vi "Trig_TimeCheck.vi"(8 "error in (no error)":errorcluster, 11 "cmd":T1) -> (0 "error out":errorcluster)   [LabVIEW 2019]
uses:
  cmd_offtimecheck.ctl
  _ctrl/system-status.ctl
  _ctrl/rw.ctl
  _ctrl/init-r-stop.ctl
  Durability/common/Global_params.vi
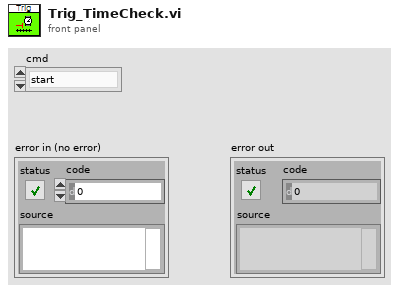
[diagram p1: front panel]
types:
  T1 = typedef "cmd_offtimecheck.ctl" = enum16{"start", "check", "init"}
  T2 = typedef "rw.ctl" = enum16{"read", "write"}
  T3 = typedef "system-status.ctl" = enum16{"Initial", "Update", "Clear", "Read"}
  T4 = typedef "init-r-stop.ctl" = enum16{"ini", "read", "stop"}
  T5 = typedef "cap_config.ctl" = cluster{"Test Mode":T6, "ON time[ms]":dbl, "OFF time[ms]":dbl, "1. 작동시간[분]":dbl, "2. 미작동시간[분]":dbl, "3. 작동시간[분]":dbl, "level[V]":dbl, "duty":dbl, "Freq":dbl, "Voltage+[V]":dbl, "Voltage-[V]":dbl, "Current+[A]":dbl, "Current-[A]":dbl, "출력전압[V]":dbl, "출력전류[A]":dbl, "OVP Level":dbl, "OCP Level":dbl, "Time Div":u16, "Record Len":i32, "방전 기준[V]":dbl, "Repeate (Each Ch)":u32, "Cycle[N]":u32, "작동간격[분]":dbl, "TrigPos[%]":dbl, "시험시간[분]":dbl}
  T6 = typedef "시험모드선택.ctl" = enum16{"6.3.1 온도방치 시험", "6.3.2 저온 작동/방치 시험", "6.3.3 고온 작동/방치 시험", "6.3.4 온도 싸이클 시험", "6.3.6 온습도 싸이클 시험", "6.3.7 고온고습 방치", "6.3.8 결로 시험", "6.3.9 빙결시험", "6.3.11.1 작동가진", "6.3.12 충격시험"}
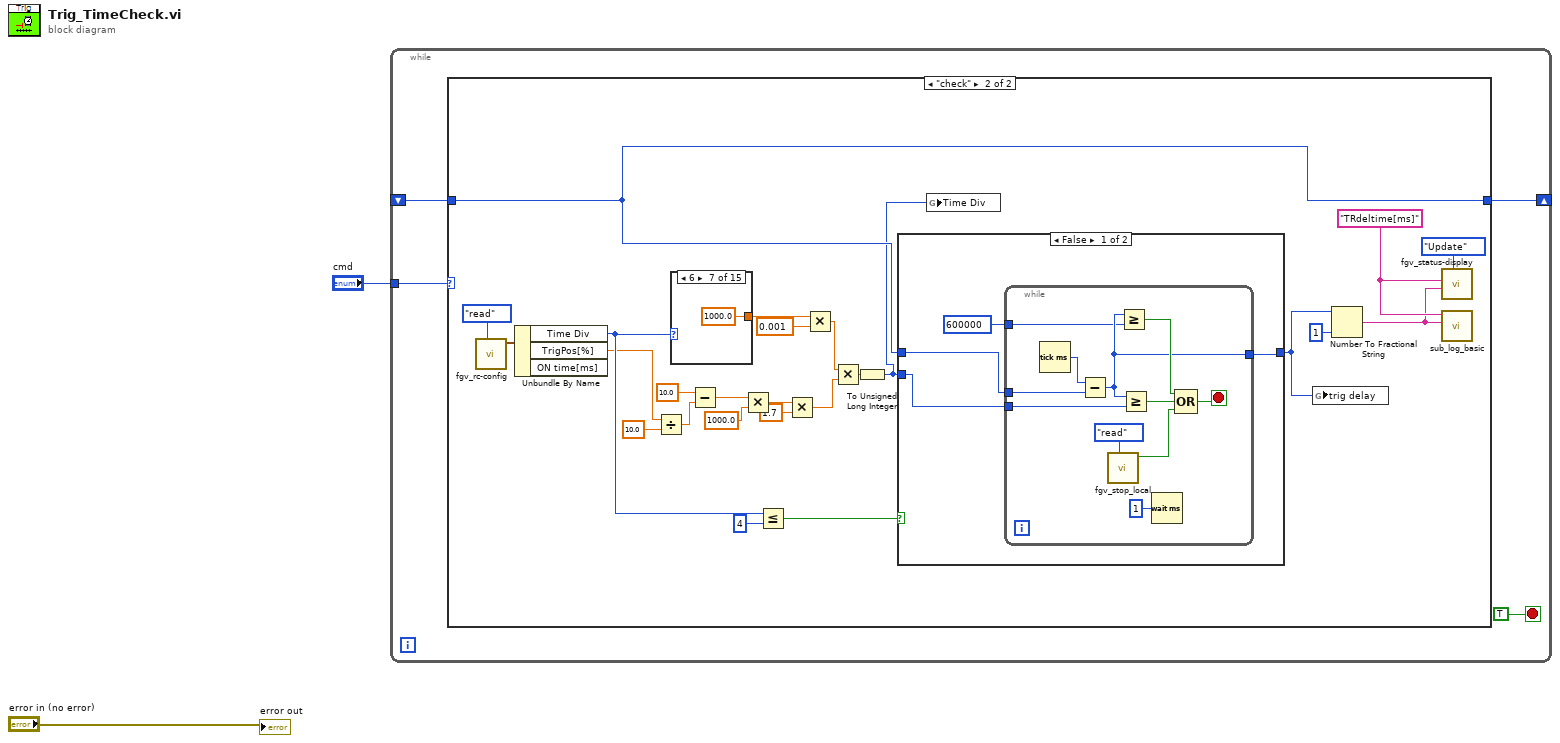
[diagram p0: block diagram]
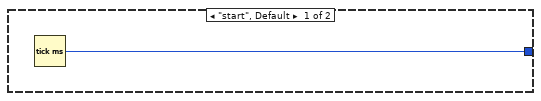
[diagram p2: hidden frame]
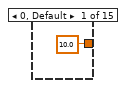
[diagram p3: hidden frame]
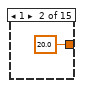
[diagram p4: hidden frame]
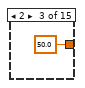
[diagram p5: hidden frame]
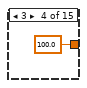
[diagram p6: hidden frame]
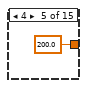
[diagram p7: hidden frame]
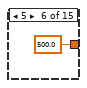
[diagram p8: hidden frame]
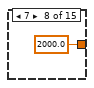
[diagram p9: hidden frame]
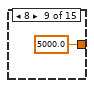
[diagram p10: hidden frame]
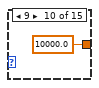
[diagram p11: hidden frame]
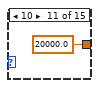
[diagram p12: hidden frame]
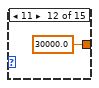
[diagram p13: hidden frame]
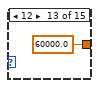
[diagram p14: hidden frame]
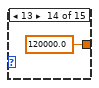
[diagram p15: hidden frame]
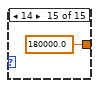
[diagram p16: hidden frame]
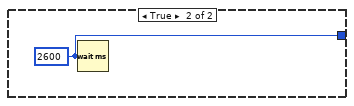
[diagram p17: hidden frame]
diagram:
  n1 = while {
    tunnel: "cmd" -> [w5]
    shift-right: [w4] -> _
    shift-left: _ -> [w3]
    stop <- TRUE stop-if-true
    n2 = case shown="\"check\"" w5 {
      tunnel: [w7 w23] -> w4
      tunnel: w3 -> [_ w23]
      frame "start", Default {
        n3 = Tick Count (ms)() -> (millisecond timer value=w7:u32)
      }
      frame "check" {
        w31 = "TRdeltime[ms]" ("title")
        n4 = call "fgv_rc-config.vi"("cmd"=rw."read") -> ("Testconfig out"=w26:T5)  [unwired: 9 in, 1 out]
        n5 = Unbundle By Name(w26) -> ("Time Div"=w19:u16, "TrigPos[%]"=w17:dbl)  [unwired: 1 out]
        n6 = Divide(x=w17, y=10.0) -> (x/y=w14:dbl)
        n7 = case shown="6" w19 {
          tunnel: [10.0 ("number") 20.0 ("number") 50.0 ("number") 100.0 ("number") 200.0 ("number") 500.0 ("number") 1000.0 ("number") 2000.0 ("number") 5000.0 ("number") 10000.0 ("number") 20000.0 ("number") 30000.0 ("number") 60000.0 ("number") 120000.0 ("number") 180000.0 ("number")] -> w21
          frame 0, Default {
          }
          frame 1 {
          }
          frame 2 {
          }
          frame 3 {
          }
          frame 4 {
          }
          frame 5 {
          }
          frame 6 {
          }
          frame 7 {
          }
          frame 8 {
          }
          frame 9 {
          }
          frame 10 {
          }
          frame 11 {
          }
          frame 12 {
          }
          frame 13 {
          }
          frame 14 {
          }
        }
        n8 = Subtract(x=10.0, y=w14) -> (x-y=w13:dbl)
        n9 = Multiply(x=w13, y=1000.0) -> (x*y=w10:dbl)
        n10 = Less Or Equal?(x=w19, y=u16 4) -> (x <= y?=w28:bool)
        n11 = Multiply(x=w10, y=1.7) -> (x*y=w8:dbl)
        n12 = Multiply(x=w21, y=0.001) -> (x*y=w18:dbl)
        n13 = Multiply(x=w18, y=w8) -> (x*y=w27:dbl)
        n14 = To Unsigned Long Integer(number=w27) -> (unsigned 32bit integer=w11:u32)
        n15 = case shown="False" w28 {
          tunnel: w11 -> [w51 _]
          tunnel: [w48 w63] -> w22
          tunnel: w23 -> [w49 _]
          frame False {
            n16 = while {
              tunnel: w49 -> [w61]
              tunnel: w51 -> [w60]
              tunnel: [w55] -> w48
              tunnel: u32 600000 ("t1") -> [w54]
              stop <- w56 stop-if-true
              n17 = Tick Count (ms)() -> (millisecond timer value=w62:u32)
              n18 = Subtract(x=w62, y=w61) -> (x-y=w55:u32)
              n19 = call "fgv_stop_local.vi"("cmd"=init-r-stop."read") -> ("stop"=w52:bool)  [unwired: 9 in, 1 out]
              n20 = Greater Or Equal?(x=w55, y=w54) -> (x >= y?=w58:bool)
              n21 = Greater Or Equal?(x=w55, y=w60) -> (x >= y?=w57:bool)
              n22 = Wait (ms)(milliseconds to wait=u32 1) -> ()  [unwired: 1 out]
              n23 = Compound Arithmetic op=OR(w58, w57, w52) -> (w56:bool)
            }
          }
          frame True {
            w63 = u32 2600 ("milliseconds to wait")
            n24 = Wait (ms)(milliseconds to wait=w63) -> ()  [unwired: 1 out]
          }
        }
        n25 = global write "Global_params.vi" "Time Div"(w11) -> ()
        n26 = global write "Global_params.vi" "trig delay"(w22) -> ()
        n27 = Number To Fractional String(number=w22, precision (6)=i16 1) -> (F-format string=w30:string)  [unwired: 2 in]
        n28 = call "fgv_status-display.vi"("Mode"=system-status."Update", "detail"=w30, "title"=w31) -> ()  [unwired: 8 in, 1 out]
        n29 = call "sub_log_basic.vi"("desc"=w30, "Title"=w31) -> ()  [unwired: 9 in, 1 out]
      }
    }
  }
  "error out" <- "error in (no error)"
